vi "Decode COB-ID.vi"(11 "COD-ID":u32 format="%.0x") -> (1 "Function Code":u8(ring) items=["NMT"=0, "EMCY/SYNC"=1, "TIME"=2, "PDO1 (tx)"=3, "PDO1 (rx)"=4, "PDO2 (tx)"=5, "PDO2 (rx)"=6, "PDO3 (tx)"=7, "PDO3 (rx)"=8, "PDO4 (tx)"=9, "PDO4 (rx)"=10, "SDO (tx)"=11, "SDO (rx)"=12, "NMT error control"=14], 3 "Node-ID":u8)   [LabVIEW 2020, in "CANopen.lvlib" / "CANopen Message.lvclass"]
uses:
  CANopen Message.lvclass
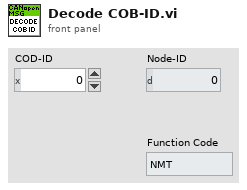
[diagram p1: front panel]
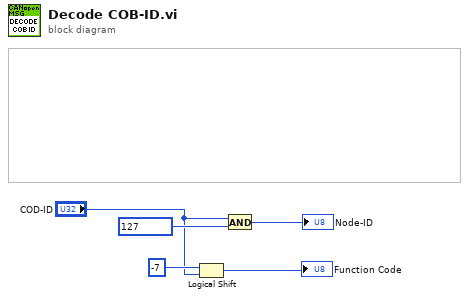
[diagram p0: block diagram]
diagram:
  n1 = Logical Shift(y=i16 -7, x="COD-ID") -> (x << y=→"Function Code":u32)
  n2 = And(x="COD-ID", y=u32 127) -> (x .and. y?=→"Node-ID":u32)
